vi "Verify Blink LE.vi"(0 "GEA2 Reference In":refnum<k24>, 1 "Standalone":bool, 2 "Blinking LED":T1, 5 "Initial Timeout (s)":dbl, 7 "Retry Count":i32, 9 "Max Blink Rate (sec)":dbl, 11 "Error In":errorcluster, 12 "Ignore Brightness":bool) -> (4 "GEA2 Reference Out":refnum<k24>, 6 "Pass/Fail?":bool, 8 "Report Text":string, 10 "Blink Times (s)":dbl[](array[numeric]), 15 "Error Out":errorcluster)   [LabVIEW 2016, in "TLMB.lvlib"]
doc: "This VI is used to verify that a particular LED is blinking on the LEUI."
uses:
  Projects/TLMB.lvlib
  Q:/Common/DLLs/GEA3/GeaCommunication.dll
  Common/DLLs/GEA3/GeaCommunication.dll
  controls/LEUI_LEDs.ctl
  Common/LabVIEW GEA2 Toolkit/LabVIEW_GEA2_Toolkit.lvlibp/type defs/Source_Destination.ctl
  Common/LabVIEW GEA2 Toolkit/LabVIEW_GEA2_Toolkit.lvlibp
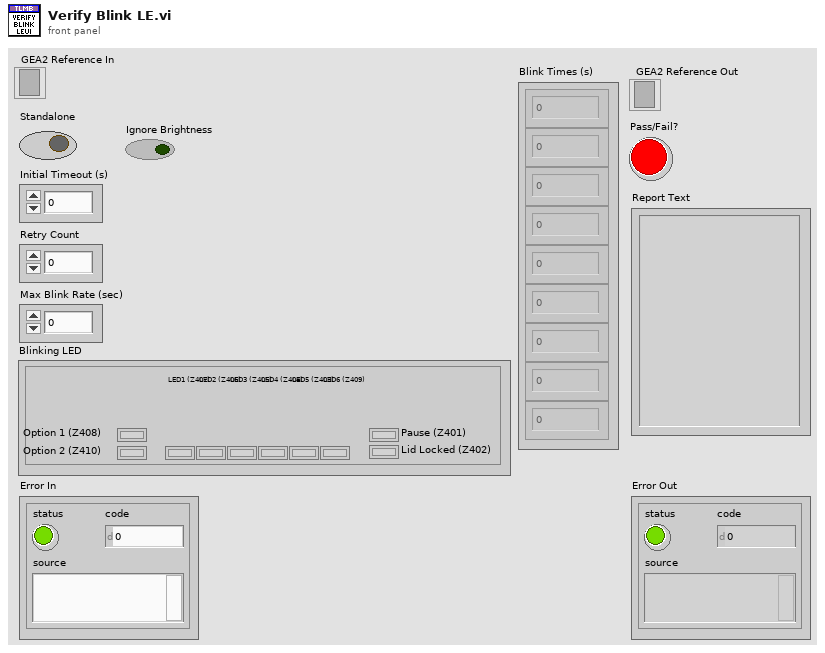
[diagram p1: front panel]
types:
  T1 = typedef "TLMB.lvlib/LEUI_LEDs.ctl" = cluster{"Pause (Z401)":bool, "Lid Locked (Z402)":bool, "LED1 (Z407)":bool, "LED2 (Z406)":bool, "LED3 (Z405)":bool, "LED4 (Z404)":bool, "LED5 (Z403)":bool, "LED6 (Z409)":bool, "Option 1 (Z408)":bool, "Option 2 (Z410)":bool}
  T2 = typedef "LabVIEW_GEA2_Toolkit.lvlibp/Source_Destination.ctl" = cluster{"Source":u8, "Destination":u8}
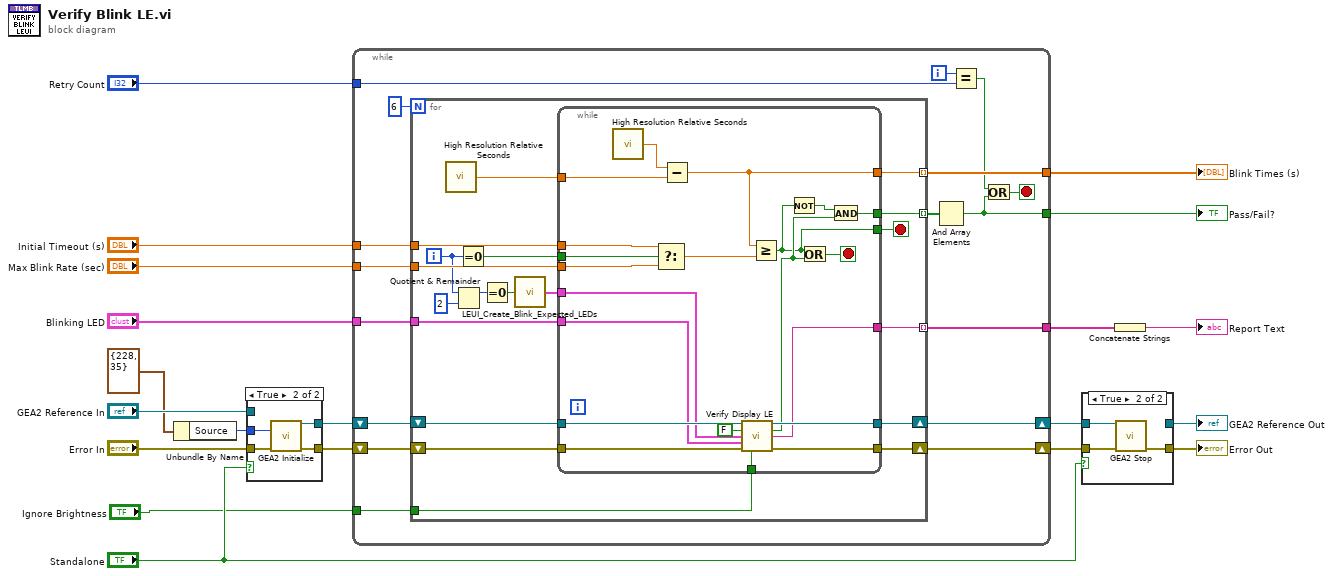
[diagram p0: block diagram]
diagram:
  n1 = Unbundle By Name(T2 {"Source"=228, "Destination"=35} ("GEA Inputs")) -> ("Source"=w19:u8)
  n2 = case shown="True" "Standalone" {
    tunnel: "Error In" -> [w22 w26]
    tunnel: w19 -> [_ w25]
    tunnel: [w21 w24] -> w11
    tunnel: [w22 w23] -> w10
    tunnel: "GEA2 Reference In" -> [w21 _]
    frame False {
    }
    frame True {
      n3 = call "GEA2 Initialize.vi"("Source Address"=w25, "error in"=w26) -> ("GEA2 Reference Out"=w24:refnum<k24>, "error out"=w23:errorcluster)  [unwired: 11 in, 1 out]
    }
  }
  n4 = while {
    tunnel: "Max Blink Rate (sec)" -> [w43]
    tunnel: [w32] -> w5
    tunnel: [w42] -> w12
    tunnel: "Blinking LED" -> [w37]
    tunnel: "Initial Timeout (s)" -> [w36]
    shift-right: [w39] -> w9
    shift-left: w11 -> [w41]
    shift-right: [w38] -> w8
    shift-left: w10 -> [w40]
    tunnel: [w35] -> w6
    tunnel: "Retry Count" -> [w29]
    tunnel: "Ignore Brightness" -> [w27]
    i -> [w30]
    stop <- w31 stop-if-true
    n5 = for {
      N: 6 -> [_]
      shift-right: [w61] -> w38
      shift-left: w40 -> [w62]
      shift-right: [w60] -> w39
      shift-left: w41 -> [w59]
      tunnel: w43 -> [w57]
      tunnel: [w55] -> w34 mode=indexing
      tunnel: [w52] -> w35 mode=indexing
      tunnel: [w56] -> w42 mode=indexing
      tunnel: w37 -> [w51]
      tunnel: w36 -> [w53]
      tunnel: w27 -> [w44]
      i -> [w45]
      stop <- w46 stop-if-true
      n6 = call <vilib>:"High Resolution Relative Seconds.vi"() -> ("relative seconds"=w58:dbl)
      n7 = Quotient & Remainder(x=w45, y=2) -> (x-y*floor(x/y)=w49:i32)  [unwired: 1 out]
      n8 = Equal To 0?(x=w45) -> (x = 0?=w54:bool)
      n9 = Equal To 0?(x=w49) -> (x = 0?=w48:bool)
      n10 = call "LEUI_Create_Blink_Expected_LEDs.vi"("Boolean"=w48) -> ("Expected LEDs Out"=w47:T1)  [unwired: 14 in]
      n11 = while {
        tunnel: w62 -> [w71]
        tunnel: [w70] -> w61
        tunnel: [w72] -> w60
        tunnel: w59 -> [w73]
        tunnel: w58 -> [w82]
        tunnel: w57 -> [w77]
        tunnel: [w80] -> w55
        tunnel: [w81] -> w56
        tunnel: w54 -> [w74]
        tunnel: w51 -> [w66]
        tunnel: w53 -> [w78]
        tunnel: [w69] -> w52
        tunnel: w47 -> [w65]
        tunnel: [w67] -> w46
        tunnel: w44 -> [w63]
        stop <- w79 stop-if-true
        n12 = call <vilib>:"High Resolution Relative Seconds.vi"() -> ("relative seconds"=w83:dbl)
        n13 = Select(t=w78, s=w74, f=w77) -> (s? t:f=w76:dbl)
        n14 = Subtract(x=w83, y=w82) -> (x-y=w81:dbl)
        n15 = call "Verify Display LE.vi"("GEA2 Reference In"=w73, "Standalone?"=FALSE, "LEUI_LEDs_Expected"=w65, "Care"=w66, "Error In"=w71, "Ignore Brightness"=w63) -> ("GEA2 Reference Out"=w72:refnum<k24>, "Pass/Fail?"=w68:bool, "Report Text"=w69:string, "Error Out"=w70:errorcluster)  [unwired: 5 in, 1 out]
        n16 = Greater Or Equal?(x=w81, y=w76) -> (x >= y?=w67:bool)
        n17 = Not(x=w67) -> (.not. x?=w75:bool)
        n18 = Or(x=w67, y=w68) -> (x .or. y?=w79:bool)
        n19 = And(x=w75, y=w68) -> (x .and. y?=w80:bool)
      }
    }
    n20 = And Array Elements(Boolean array=w34) -> (logical AND=w32:bool)
    n21 = Equal?(x=w30, y=w29) -> (x = y?=w33:bool)
    n22 = Or(x=w33, y=w32) -> (x .or. y?=w31:bool)
  }
  "Pass/Fail?" <- w5
  "Blink Times (s)" <- w12
  n23 = case shown="True" "Standalone" {
    tunnel: w8 -> [w85 w88]
    tunnel: [w85 w87] -> w17
    tunnel: w9 -> [w84 w86]
    tunnel: [w84 _] -> w15
    frame False {
    }
    frame True {
      n24 = call "GEA2 Stop.vi"("GEA2 Reference In"=w86, "Error In"=w88) -> ("Error Out"=w87:errorcluster)  [unwired: 13 in]
    }
  }
  "GEA2 Reference Out" <- w15
  "Error Out" <- w17
  n25 = Concatenate Strings(w6) -> (→"Report Text":string)
